vi "UploadIV.vi"(8 "UiDefinition 2":T1, 9 "Cluster":T2, 10 "IV Scan Data":dbl[][](array[numeric]), 11 "url":string) -> ()   [LabVIEW 2020]
uses:
  UIReferences.ctl
  D:/LabviewDXFViewer/LabviewDXFViewer/bin/Release/LabviewDXFViewer.exe
  LabviewDXFViewer/bin/Release/LabviewDXFViewer.exe
  <vilib>/httpClient/POSTBuffer.vi
  <vilib>/httpClient/LabVIEWHTTPClient.lvlib
panel:
  out "error out":errorcluster
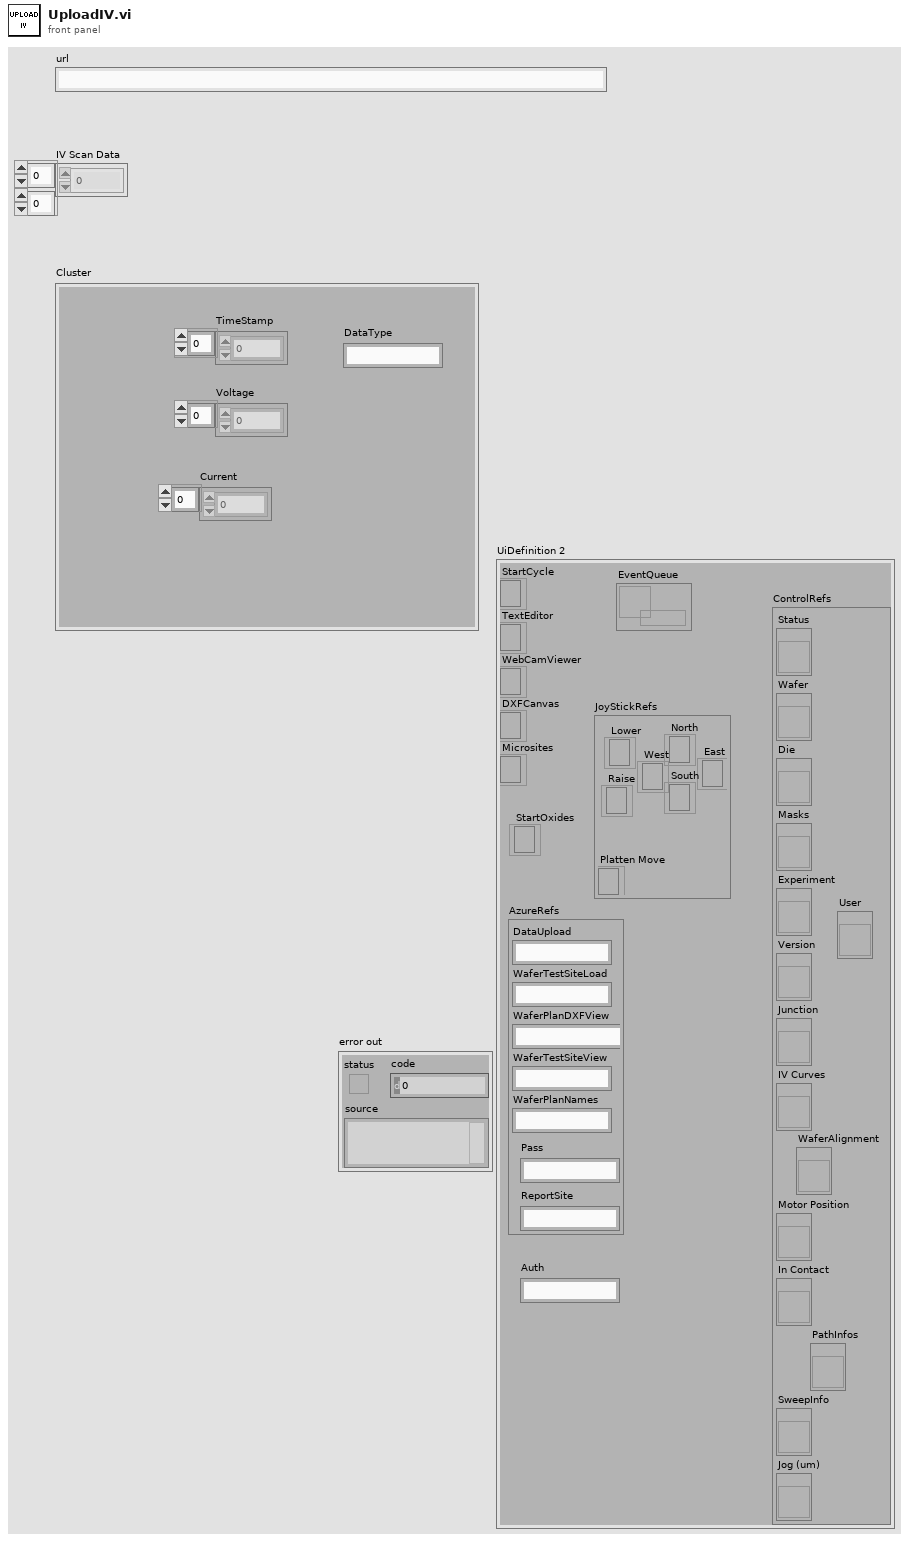
[diagram p1: front panel]
types:
  T1 = typedef "UIReferences.ctl" = cluster{"StartCycle":refnum<k24>, "TextEditor":refnum<k24>, "WebCamViewer":refnum<k24>, "DXFCanvas":refnum<k24>, "Microsites":refnum<k24>, "JoyStickRefs":cluster{"North":refnum<k24>, "Lower":refnum<k24>, "Raise":refnum<k24>, "Platten Move":refnum<k24>, "West":refnum<k24>, "East":refnum<k24>, "South":refnum<k24>}, "AzureRefs":cluster{"DataUpload":string, "WaferTestSiteLoad":string, "WaferPlanDXFView":string, "WaferTestSiteView":string, "WaferPlanNames":string, "Pass":string, "ReportSite":string}, "ControlRefs":cluster{"Status":refnum<vi>, "Wafer":refnum<vi>, "Die":refnum<vi>, "Masks":refnum<vi>, "Experiment":refnum<vi>, "Version":refnum<vi>, "Junction":refnum<vi>, "IV Curves":refnum<vi>, "Motor Position":refnum<vi>, "In Contact":refnum<vi>, "SweepInfo":refnum<vi>, "Jog (um)":refnum<vi>, "PathInfos":refnum<vi>, "User":refnum<vi>, "WaferAlignment":refnum<vi>}, "EventQueue":refnum<queue>, "StartOxides":refnum<k24>, "Auth":string}
  T2 = cluster{"TimeStamp":dbl[], "Voltage":dbl[], "Current":dbl[], "DataType":string}
  T3 = typedef "LabVIEWHTTPClient.lvlib/ClientHandle.ctl" = refnum<k1>
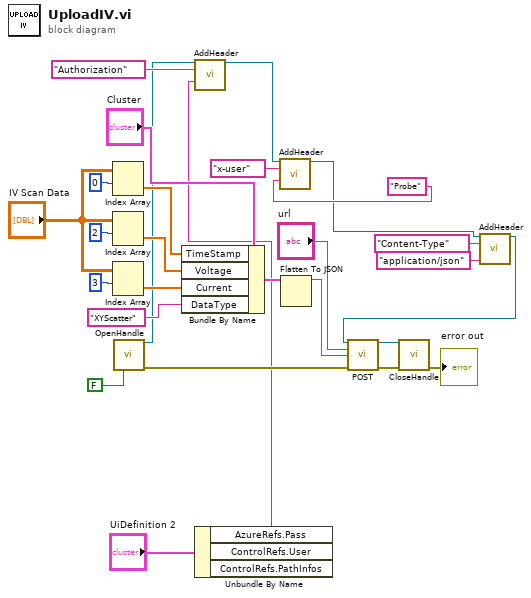
[diagram p0: block diagram]
diagram:
  n1 = Index Array(array="IV Scan Data", index (row)=0) -> (element=w20:dbl[])  [unwired: 1 in]
  n2 = Index Array(array="IV Scan Data", index (row)=2) -> (element=w23:dbl[])  [unwired: 1 in]
  n3 = Index Array(array="IV Scan Data", index (row)=3) -> (element=w24:dbl[])  [unwired: 1 in]
  n4 = call <vilib>:"OpenHandle.vi"("verify server(true)"=FALSE) -> ("client handle out"=w8:T3, "error out"=w16:errorcluster)  [unwired: 13 in]
  n5 = Bundle By Name(cluster="Cluster", "TimeStamp"=w20, "Voltage"=w23, "Current"=w24, "DataType"="XYScatter") -> (w25:T2)
  n6 = Unbundle By Name("UiDefinition 2") -> ("AzureRefs.Pass"=w6:string)  [unwired: 2 out]
  n7 = call <vilib>:"AddHeader.vi"("client handle"=w8, "header"="Authorization", "value"=w6) -> ("client handle out"=w11:T3)  [unwired: 11 in, 1 out]
  n8 = call <vilib>:"AddHeader.vi"("client handle"=w11, "header"="x-user", "value"="Probe") -> ("client handle out"=w4:T3)  [unwired: 11 in, 1 out]
  n9 = Flatten To JSON(anything=w25) -> (JSON string=w18:string)  [unwired: 2 in, 1 out]
  n10 = call <vilib>:"AddHeader.vi"("client handle"=w4, "header"="Content-Type", "value"="application/json") -> ("client handle out"=w3:T3)  [unwired: 11 in, 1 out]
  n11 = call-poly <vilib>:"POST.vi"("client handle"=w3, "url"="url", "buffer"=w18, "error in (no error)"=w16) -> ("client handle out"=w28:T3, "error out"=w17:errorcluster)  [unwired: 8 in, 2 out]
  n12 = call <vilib>:"CloseHandle.vi"("client handle"=w28, "error in (no error)"=w17) -> ("error out"=→"error out":errorcluster)  [unwired: 13 in]
